vi "Save JPG Image (Core).vi"(8 "error in (no error)":errorcluster, 9 "Quality (85)":i32=85, 10 "Picture":T1, 11 "Path In":string) -> (0 "error out":errorcluster, 3 "Path Out":string)   [LabVIEW 2020, in "G-Image.lvlib"]
doc: "Retrieve audio file information. Some codecs (mp3) require the entire file be parsed to accurately determine the length, which can take time for very large files.\n\nSupported codecs: flac, mp3, ogg (vorbis), and wav."
uses:
  G-Image.lvlib
  <vilib>/picture/picture.llb/imagedata.ctl
  Controls/Image Save Format.ctl
  Private/ARGB To RGBA.vi
  <vilib>/Utility/file.llb/Application Directory.vi
  <vilib>/Utility/error.llb/Error Cluster From Error Code.vi
  lib/g_image_32.dll
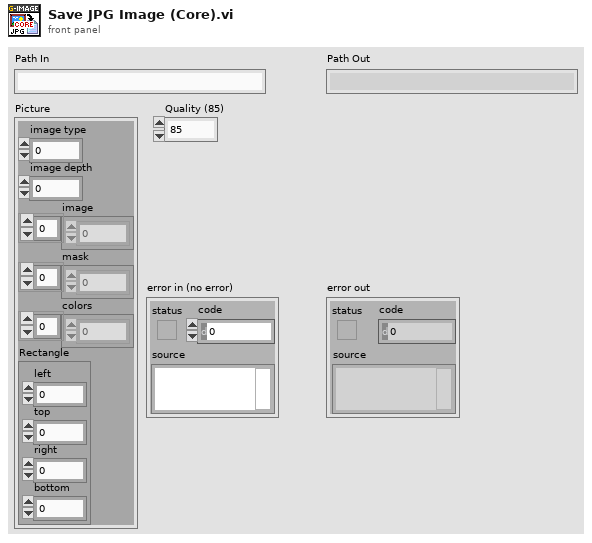
[diagram p1: front panel]
types:
  T1 = typedef "imagedata.ctl" = cluster{"image type":i32, "image depth":i32, "image":u8[], "mask":u8[], "colors":u32[], "Rectangle":cluster{"left":i16, "top":i16, "right":i16, "bottom":i16}}
  T2 = typedef "G-Image.lvlib/Image Save Format.ctl" = enum16{"png", "jpg", "bmp", "gif", "tga"}
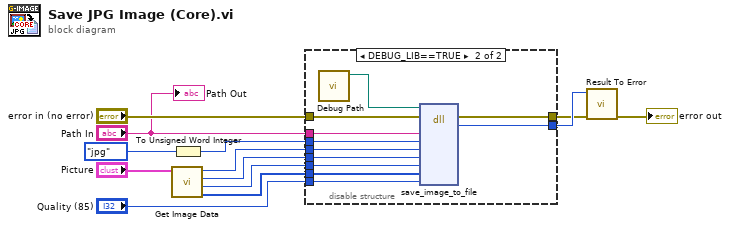
[diagram p0: block diagram]
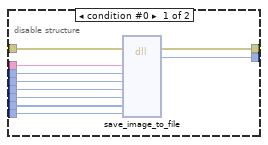
[diagram p2: hidden frame]
diagram:
  n1 = call "Get Image Data.vi"("Image"="Picture") -> ("Image (RGBA)"=w2:u8[], "Channels"=w3:i32, "Height"=w4:i32, "Width"=w5:i32)  [unwired: 7 in]
  n2 = To Unsigned Word Integer(number=Image_Save_Format."jpg" ("Save Format")) -> (unsigned 16bit integer=w8:u16)
  n3 = disable-structure shown="DEBUG_LIB==TRUE" {
    disable-tunnel: [w23 w34] -> w11
    disable-tunnel: "error in (no error)" -> [w22 w33]
    disable-tunnel: "Path In" -> [w21 w32]
    disable-tunnel: [w20 w31] -> w12
    disable-tunnel: w8 -> [w19 w30]
    disable-tunnel: w5 -> [w18 w29]
    disable-tunnel: w4 -> [w17 w28]
    disable-tunnel: w3 -> [w16 w27]
    disable-tunnel: w2 -> [w15 w26]
    disable-tunnel: "Quality (85)" -> [w14 w24]
    frame condition #0 {
      n4 = dll-call lib="C:/github/dataflowg/g-image/src/LabVIEW/G-Image/lib/g_image_*.*" fn="save_image_to_file"(error in=w22, "file_name"=w21, "format"=w19, "width"=w18, "height"=w17, "channels"=w16, "image_data"=w15, "option"=w14) -> (error out=w23:errorcluster, "result"=w20:i32)  [unwired: 9 in, 1 out]
    }
    frame condition #1 (active) {
      n5 = call "Debug Path.vi"() -> ("Debug Path"=w25:path)  [unwired: 11 in]
      n6 = dll-call lib="?" fn="save_image_to_file"(path in=w25, error in=w33, "file_name"=w32, "format"=w30, "width"=w29, "height"=w28, "channels"=w27, "image_data"=w26, "option"=w24) -> (error out=w34:errorcluster, "result"=w31:i32)  [unwired: 8 in, 1 out]
    }
  }
  n7 = call "Result To Error.vi"("error in (no error)"=w11, "Result Code"=w12) -> ("error out"=→"error out":errorcluster)  [unwired: 9 in]
  "Path Out" <- "Path In"
